vi "SetClassCtrl.vi"(8 "error in (no error)":errorcluster caption="entrée d'erreur (pas d'erreur)", 10 "ClassCtrlRef":refnum<vi>, 11 "PhotoLum en entrée":refnum<class "PhotoLum.lvclass"> caption="DNL_LabVIEW Object in") -> (0 "error out":errorcluster caption="sortie d'erreur", 3 "PhotoLum en sortie":refnum<class "PhotoLum.lvclass"> caption="DNL_LabVIEW Object out")   [LabVIEW 2019, in "PhotoLum.lvclass"]
uses:
  PhotoLum.lvclass
  BaseDevice/BaseDevice.lvclass
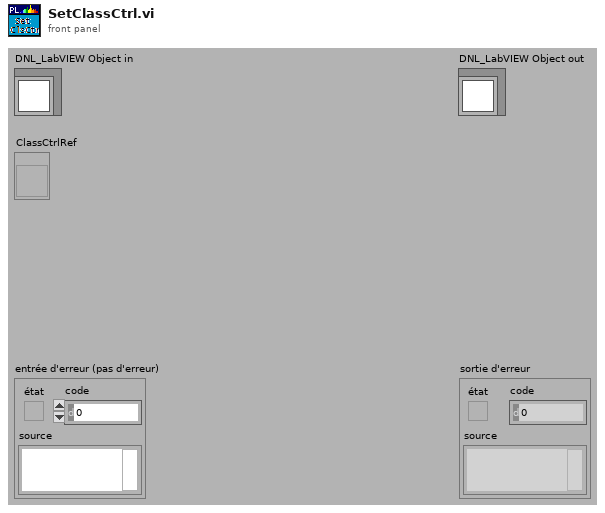
[diagram p1: front panel]
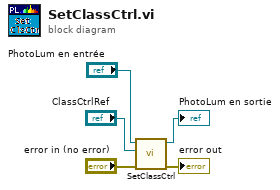
[diagram p0: block diagram]
diagram:
  n1 = call-parent "SetClassCtrl.vi"("error in (no error)"="error in (no error)", "ClassCtrlRef"="ClassCtrlRef", "BaseDevice en entrée"="PhotoLum en entrée") -> ("error out"=→"error out":errorcluster, "BaseDevice en sortie"=→"PhotoLum en sortie":refnum<class "PhotoLum.lvclass">)  [unwired: 7 in]
